vi "Flow_spiderplot.vi"(3 "error in":errorcluster, 5 "3XNSensors":dbl[][](array[numeric])) -> (0 "error out":errorcluster, 1 "new picture":picture)   [LabVIEW 2013]
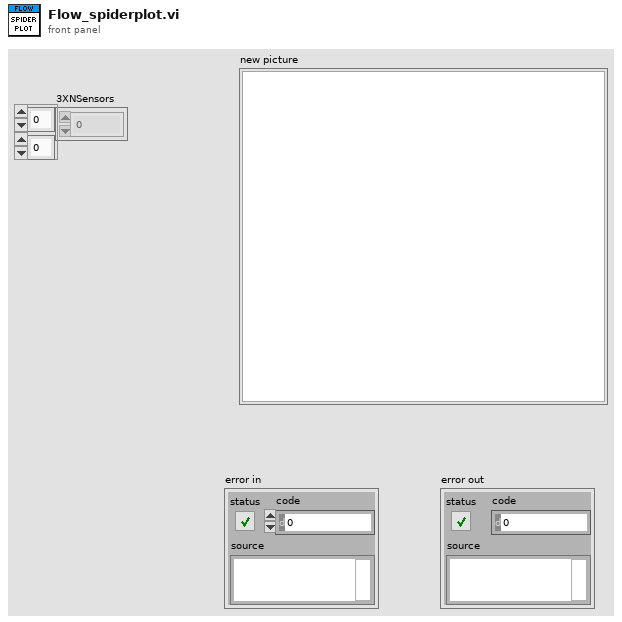
[diagram p1: front panel]
types:
  T1 = cluster{"plot name":string, "color (white)":u32, "fill?(F)":bool}[]
  T2 = cluster{"color (white)":u32, "format and precision":cluster{"format":enum8{"Decimal", "Scientific", "Engineering", "Binary", "Octal", "Hex"}, "precision":u8}, "autoscale? (false)":bool}
  T3 = cluster{"label":string, "max value":dbl, "min value":dbl}[]
  T4 = enum16{"User-specified Font", "Application Font", "System Font", "Dialog Font"}
  T5 = cluster{"Font Name:":string, "Size":i16, "Strikeout?":bool, "Italic?":bool, "Underline?":bool, "Outline?":bool, "Shadow?":bool, "Bold?":bool}
  T6 = cluster{"position (none)":enum16{"none", "top", "right", "bottom", "left"}, "text color(white)":u32}
  T7 = cluster{"x":i16, "y":i16, "Width":i16, "Width":i16}
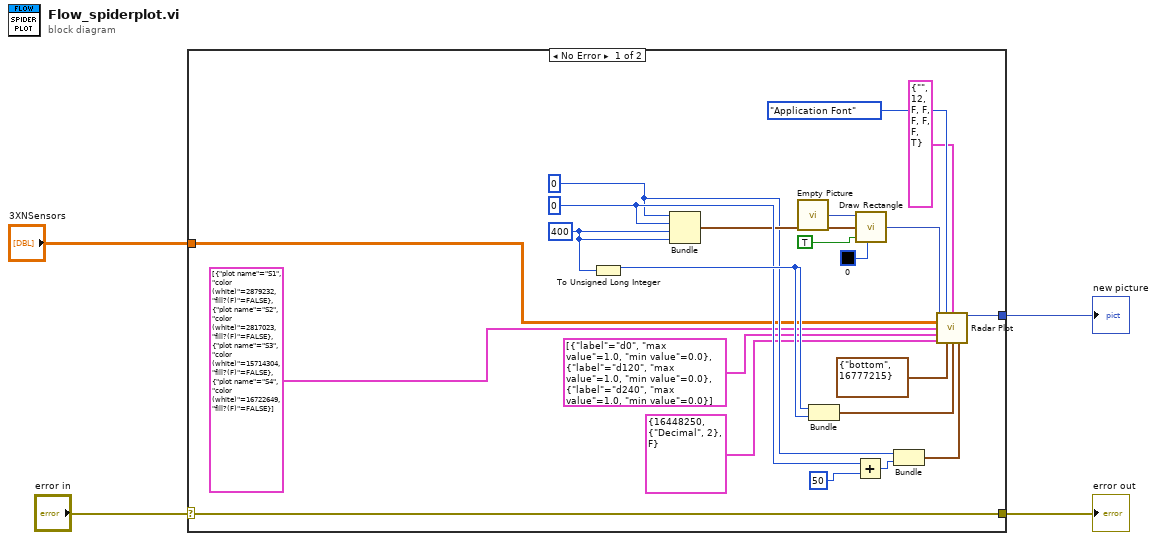
[diagram p0: block diagram]
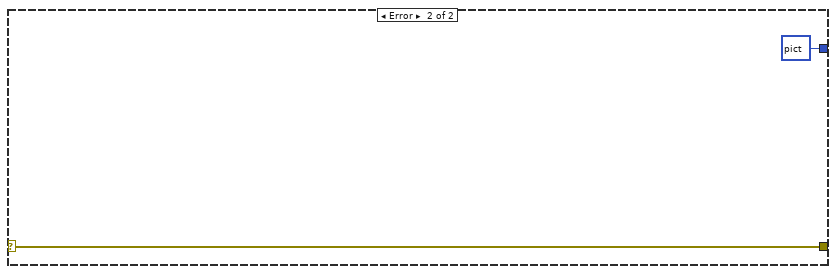
[diagram p2: hidden frame]
diagram:
  n1 = case shown="No Error" "error in" {
    selector: "error in" -> [w7 w27]
    tunnel: [w8 picture data[5B] ("new picture")] -> w4
    tunnel: [w7 w27] -> w2
    tunnel: "3XNSensors" -> [w5 _]
    frame No Error {
      w25 = i16 400 ("Width")
      w20 = i16 0 ("x")
      w23 = i16 0 ("y")
      n2 = To Unsigned Long Integer(number=w25) -> (unsigned 32bit integer=w26:u32)
      n3 = Bundle("x"=w20, "y"=w23, "Width"=w25, "Width"=w25) -> (w21:T7)  [unwired: 1 in]
      n4 = call "Empty Picture"() -> ("empty picture"=w15:picture)
      n5 = Bundle(w26, w26) -> (w18:cluster{u32, u32})  [unwired: 1 in]
      n6 = Add(x=w23, y=i16 50 ("Width")) -> (x+y=w24:i16)
      n7 = call <vilib>:"Draw Rectangle.vi"("picture"=w15, "rect"=w21, "fill?(F)"=TRUE, "color(black)"=u32 0) -> ("new picture"=w17:picture)  [unwired: 5 in]
      n8 = Bundle("x"=w20, w24) -> (w19:cluster{"x":i16, i16})  [unwired: 1 in]
      n9 = call <vilib>:"Radar Plot.vi"("picture"=w17, "desired font(Application)"=T4."Application Font", "[user-specified font]"=T5 {"Font Name:"="", "Size"=12, "Strikeout?"=FALSE, "Italic?"=FALSE, "Underline?"=FALSE, "Outline?"=FALSE, "Shadow?"=FALSE, "Bold?"=TRUE}, "data"=w5, "plot info"=T1 [{"plot name"="S1", "color (white)"=2879232, "fill?(F)"=FALSE}, {"plot name"="S2", "color (white)"=2817023, "fill?(F)"=FALSE}, {"plot name"="S3", "color (white)"=15714304, "fill?(F)"=FALSE}, {"plot name"="S4", "color (white)"=16722649, "fill?(F)"=FALSE}] ("Sensors"), "axis info"=T3 [{"label"="d0", "max value"=1.0, "min value"=0.0}, {"label"="d120", "max value"=1.0, "min value"=0.0}, {"label"="d240", "max value"=1.0, "min value"=0.0}], "axes info"=T2 {"color (white)"=16448250, "format and precision"={"format"=enum."Decimal", "precision"=2}, "autoscale? (false)"=FALSE}, "legend info"=T6 {"position (none)"=enum."bottom", "text color(white)"=16777215}, "dimension (w,h)"=w18, "top left point(0, 0)"=w19) -> ("new picture"=w8:picture)  [unwired: 5 in]
    }
    frame Error {
    }
  }
  "new picture" <- w4
  "error out" <- w2
